vi "handler_results.vi"(8 "error in (no error)":errorcluster, 10 "Server Variables":T1 {"Energy Levels"."E1" format="%_6g"; "Phases"."ExtTriggerDelay" format="%.3g"}, 11 "HTTP Request in":T7) -> (0 "error out":errorcluster, 2 "Server Variables":T1 {"Energy Levels"."E1" format="%_6g"; "Phases"."ExtTriggerDelay" format="%.3g"}, 3 "HTTP Request out":T7)   [LabVIEW 2011]
uses:
  http_request_response.ctl
  http_request.ctl
  http_field.ctl
  http_response.ctl
  template_field.ctl
  template_field_type.ctl
  Server Variables.ctl
  Phase Parameters.ctl
  Phase Mode.ctl
  Energy Level_.ctl
  Measurement Parameters.ctl
  Results.ctl
  JSON BDP Result.ctl
panel:
  in  "Energy discretisation":dbl=2.0
  in  "BD Threshold":dbl=0.06
  out "concatenated string":string
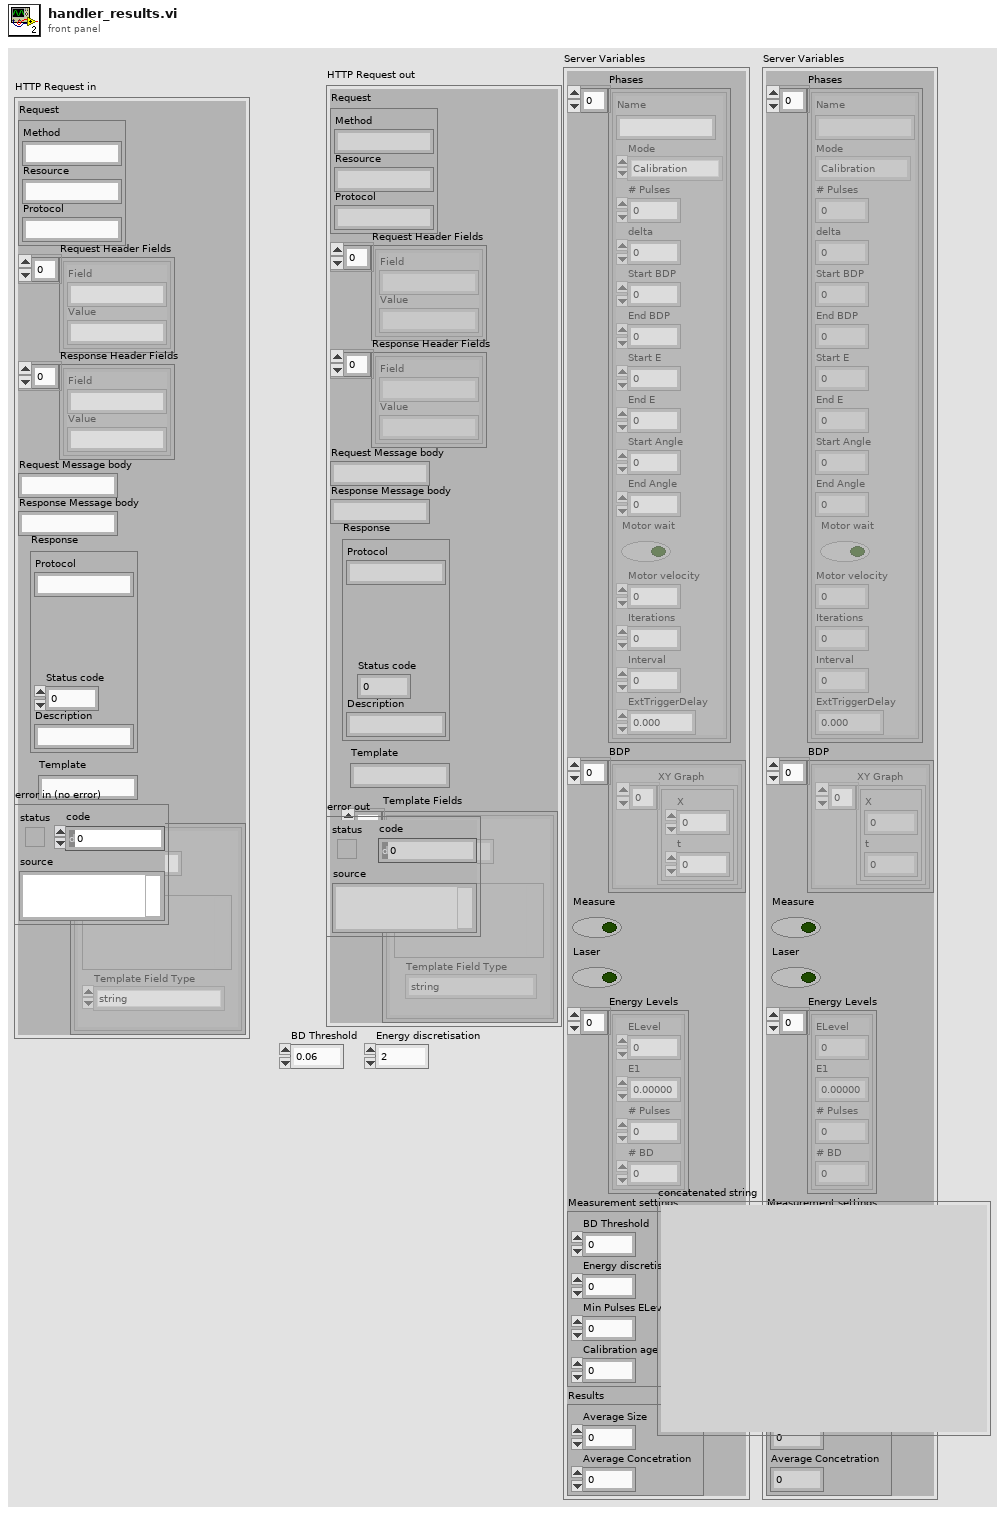
[diagram p1: front panel]
types:
  T1 = typedef "Server Variables.ctl" = cluster{"Phases":T2[], "BDP":cluster{"XY Graph":cluster{"X":dbl, "t":dbl}[]}[], "Measure":bool, "Laser":bool, "Energy Levels":T4[], "Measurement settings":T5, "Results":T6}
  T2 = typedef "Phase Parameters.ctl" = cluster{"Name":string, "Mode":T3, "# Pulses":u32, "delta":dbl, "Start BDP":dbl, "End BDP":dbl, "Start E":dbl, "End E":dbl, "Start Angle":dbl, "End Angle":dbl, "Motor wait":bool, "Motor velocity":dbl, "Iterations":dbl, "Interval":dbl, "ExtTriggerDelay":dbl}
  T3 = typedef "Phase Mode.ctl" = enum16{"Calibration", "Linear", "BDP-Fit", "Raw"}
  T4 = typedef "Energy Level_.ctl" = cluster{"ELevel":dbl, "E1":dbl, "# Pulses":i32, "# BD":i32}
  T5 = typedef "Measurement Parameters.ctl" = cluster{"BD Threshold":dbl, "Energy discretisation":i32, "Min Pulses ELevel":i32, "Calibration age":i32}
  T6 = typedef "Results.ctl" = cluster{"Average Size":dbl, "Average Concetration":dbl}
  T7 = typedef "http_request_response.ctl" = cluster{"Request":T8, "Request Header Fields":T9[], "Response Header Fields":T9[], "Request Message body":string, "Response Message body":string, "Response":T10, "Template":string, "Template Fields":T11[]}
  T8 = typedef "http_request.ctl" = cluster{"Method":string, "Resource":string, "Protocol":string}
  T9 = typedef "http_field.ctl" = cluster{"Field":string, "Value":string}
  T10 = typedef "http_response.ctl" = cluster{"Protocol":string, "Status code":dbl, "Description":string}
  T11 = typedef "template_field.ctl" = cluster{"Name":string, "Template Field Type":T12, "data":variant}
  T12 = typedef "template_field_type.ctl" = enum16{"string", "string array", "number", "number array", "cluster", "cluster array"}
  T13 = typedef "JSON BDP Result.ctl" = cluster{"bdp":cluster{"E":dbl, "BDP":dbl}[], "diameter":dbl, "concentration":dbl}
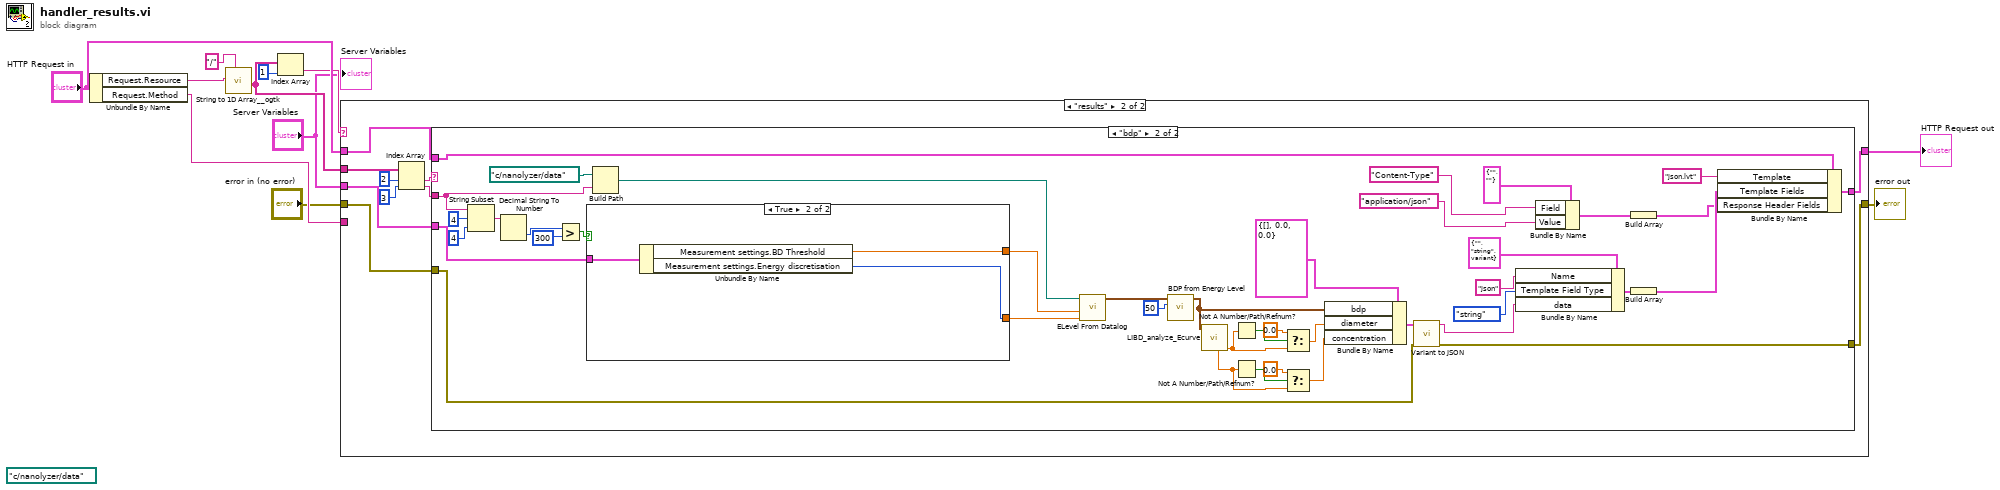
[diagram p0: block diagram]
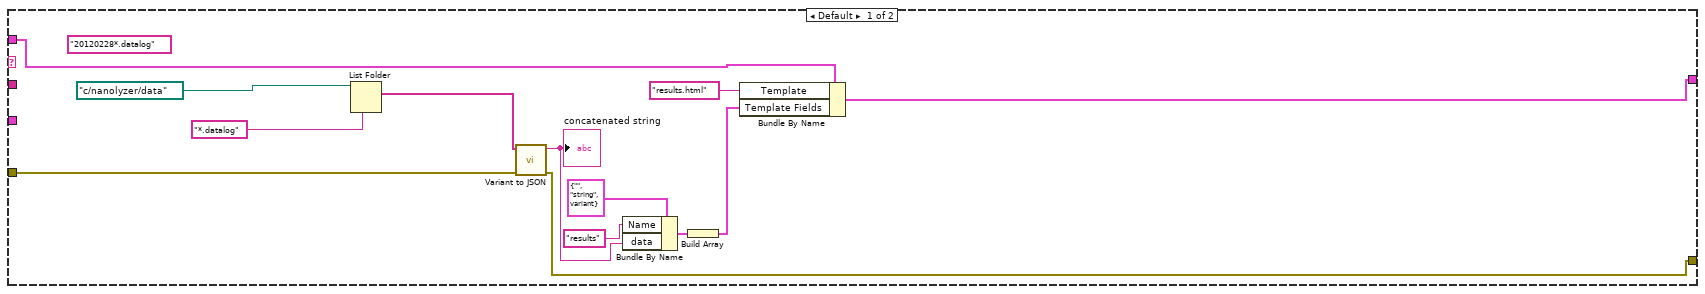
[diagram p3: hidden frame]
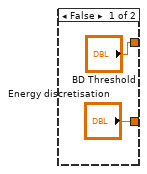
[diagram p4: hidden frame]
diagram:
  (unwired) path "c:/nanolyzer/data" ("path")
  n1 = Unbundle By Name("HTTP Request in") -> ("Request.Resource"=w6:string, "Request.Method"=w11:string)
  n2 = call <userlib>:"String to 1D Array__ogtk.vi"("delimiter (Tab)"="/", "string"=w6) -> ("Array of Strings"=w2:string[])  [unwired: 9 in]
  n3 = Index Array(array=w2, index=1) -> (element=w3:string)
  n4 = case shown="\"results\"" w3 {
    tunnel: w11 -> [_ _]
    tunnel: "HTTP Request in" -> [w13 w18]
    tunnel: [w13 w17] -> w9
    tunnel: "error in (no error)" -> [w12 w16]
    tunnel: [w12 w15] -> w7
    tunnel: w2 -> [_ w21]
    tunnel: "Server Variables" -> [_ w14]
    frame Default {
    }
    frame "results" {
      n5 = Index Array(array=w21, index #1=2 ("index"), index #2=3 ("index")) -> (element #1=w20:string, element #2=w19:string)
      n6 = case shown="\"bdp\"" w20 {
        tunnel: w19 -> [_ w54]
        tunnel: w18 -> [w36 w76]
        tunnel: [w35 w77] -> w17
        tunnel: w16 -> [w28 w63]
        tunnel: [w27 w62] -> w15
        tunnel: w14 -> [_ w45]
        frame Default {
          (unwired) "20120228*.datalog" ("pattern")
          n7 = List Folder(path=path "c:/nanolyzer/data", pattern="*.datalog") -> (filenames=w25:string[])  [unwired: 2 in, 3 out]
          n8 = call "Variant to JSON.vi"("error in"=w28, "variant"=w25) -> ("error out"=w27:errorcluster, "concatenated string"=w29:string)  [unwired: 8 in]
          "concatenated string" <- w29
          n9 = Bundle By Name(cluster=T11 {"Name"="", "Template Field Type"=enum."string", "data"=variant} ("Template Field"), "Name"="results", "data"=w29) -> (w31:T11)
          n10 = Build Array(w31) -> (w32:T11[])
          n11 = Bundle By Name(cluster=w36, "Template"="results.html", "Template Fields"=w32) -> (w35:T7)
        }
        frame "bdp" {
          n12 = String Subset(string=w54, offset (0)=4, length (rest)=4 ("length (rest)")) -> (substring=w51:string)
          n13 = Decimal String To Number(string=w51) -> (number=w50:i32)  [unwired: 2 in, 1 out]
          n14 = Greater?(x=w50, y=300) -> (0:w46:bool)
          n15 = case shown="True" w46 {
            tunnel: ["BD Threshold" w81] -> w48
            tunnel: ["Energy discretisation" w80] -> w47
            tunnel: w45 -> [_ w82]
            frame False {
            }
            frame True {
              n16 = Unbundle By Name(w82) -> ("Measurement settings.BD Threshold"=w81:dbl, "Measurement settings.Energy discretisation"=w80:i32)
            }
          }
          n17 = Build Path(base path=path "c:/nanolyzer/data" ("path"), name or relative path=w54) -> (appended path=w60:path)
          n18 = call "ELevel From Datalog.vi"("Energy discretisation"=w47, "BD Threshold"=w48, "appended path"=w60) -> ("Energy Levels out"=w56:T4[])  [unwired: 5 in, 3 out]
          n19 = call "BDP from Energy Level.vi"("# Pulse / Energy Level Threshold"=50, "Energy Levels"=w56) -> ("BDP"=w55:cluster{"X":dbl, "Y":dbl}[])  [unwired: 9 in]
          n20 = call "LIBD_analyze_Ecurve.vi"("BDP out 2"=w55) -> ("diameter"=w40:dbl, "concentration"=w39:dbl)  [unwired: 5 in, 4 out]
          n21 = Not A Number/Path/Refnum?(number/path/refnum=w40) -> (NaN/Path/Refnum?=w44:bool)
          n22 = Not A Number/Path/Refnum?(number/path/refnum=w39) -> (NaN/Path/Refnum?=w41:bool)
          n23 = Select(t=0.0, s=w44, f=w40) -> (s? t:f=w37:dbl)
          n24 = Select(t=0.0, s=w41, f=w39) -> (s? t:f=w38:dbl)
          n25 = Bundle By Name(cluster=T13 {"bdp"=[], "diameter"=0.0, "concentration"=0.0}, "bdp"=w55, "diameter"=w37, "concentration"=w38) -> (w58:T13)
          n26 = call "Variant to JSON.vi"("error in"=w63, "variant"=w58) -> ("error out"=w62:errorcluster, "concatenated string"=w70:string)  [unwired: 8 in]
          n27 = Bundle By Name(cluster=T11 {"Name"="", "Template Field Type"=enum."string", "data"=variant} ("Template Field"), "Name"="json", "Template Field Type"=template_field_type."string", "data"=w70) -> (w66:T11)
          n28 = Bundle By Name(cluster=T9 {"Field"="", "Value"=""} ("Header Field"), "Field"="Content-Type", "Value"="application/json") -> (w72:T9)
          n29 = Build Array(w72) -> (w64:T9[])
          n30 = Build Array(w66) -> (w65:T11[])
          n31 = Bundle By Name(cluster=w76, "Template"="json.lvt", "Template Fields"=w65, "Response Header Fields"=w64) -> (w77:T7)
        }
      }
    }
  }
  "HTTP Request out" <- w9
  "error out" <- w7
  "Server Variables" <- "Server Variables"
